vi "Methods_Insert Dividers.vi"(11 "Methods[] In":T1(array[cluster])) -> (3 "Methods[] Out":T1(array[cluster]))   [LabVIEW 2023] (continued)
"Data name"="License.Get Feature Status", "Short name (localized)"="License.Get Feature Status", "Long name (localized)"="License:Get Feature Status"}, "Method Flags"={"IsDeprecated"=FALSE, "IsPrivate"=TRUE, "IsScripting"=FALSE, "IsNotInRun-Time"=FALSE}, "Divider"=FALSE}, {"Class Info"={"Unique ID string"="1", "Parent ID string"="", "Class Name (unlocalized)"="Application", "Class Name (localized)"="Application"}, "Method Info"={"Unique ID string"="849", "Data name"="Library.Deploy Library", "Short name (localized)"="Library.Deploy Library", "Long name (localized)"="Library:Deploy Library"}, "Method Flags"={"IsDeprecated"=FALSE, "IsPrivate"=FALSE, "IsScripting"=FALSE, "IsNotInRun-Time"=FALSE}, "Divider"=FALSE}, {"Class Info"={"Unique ID string"="1", "Parent ID string"="", "Class Name (unlocalized)"="Application", "Class Name (localized)"="Application"}, "Method Info"={"Unique ID string"="84b", "Data name"="NI Sec.ChangePassword", "Short name (localized)"="NI Sec.ChangePassword", "Long name (localized)"="NI Security:Change Password"}, "Method Flags"={"IsDeprecated"=FALSE, "IsPrivate"=TRUE, "IsScripting"=FALSE, "IsNotInRun-Time"=FALSE}, "Divider"=FALSE}, {"Class Info"={"Unique ID string"="1", "Parent ID string"="", "Class Name (unlocalized)"="Application", "Class Name (localized)"="Application"}, "Method Info"={"Unique ID string"="84c", "Data name"="NI Sec.GetDomains", "Short name (localized)"="NI Sec.GetDomains", "Long name (localized)"="NI Security:Get Domains"}, "Method Flags"={"IsDeprecated"=FALSE, "IsPrivate"=TRUE, "IsScripting"=FALSE, "IsNotInRun-Time"=FALSE}, "Divider"=FALSE}, {"Class Info"={"Unique ID string"="1", "Parent ID string"="", "Class Name (unlocalized)"="Application", "Class Name (localized)"="Application"}, "Method Info"={"Unique ID string"="84d", "Data name"="Save Stock Objects", "Short name (localized)"="Save Stock Objects", "Long name (localized)"="Save Stock Objects"}, "Method Flags"={"IsDeprecated"=FALSE, "IsPrivate"=TRUE, "IsScripting"=FALSE, "IsNotInRun-Time"=TRUE}, "Divider"=FALSE}, {"Class Info"={"Unique ID string"="1", "Parent ID string"="", "Class Name (unlocalized)"="Application", "Class Name (localized)"="Application"}, "Method Info"={"Unique ID string"="84e", "Data name"="Library.UndeployLibrary", "Short name (localized)"="Library.UndeployLibrary", "Long name (localized)"="Library:Undeploy Library"}, "Method Flags"={"IsDeprecated"=FALSE, "IsPrivate"=FALSE, "IsScripting"=FALSE, "IsNotInRun-Time"=FALSE}, "Divider"=FALSE}, {"Class Info"={"Unique ID string"="1", "Parent ID string"="", "Class Name (unlocalized)"="Application", "Class Name (localized)"="Application"}, "Method Info"={"Unique ID string"="84f", "Data name"="Cmp Data Types", "Short name (localized)"="Cmp Data Types", "Long name (localized)"="Compare:Data Types"}, "Method Flags"={"IsDeprecated"=FALSE, "IsPrivate"=TRUE, "IsScripting"=FALSE, "IsNotInRun-Time"=FALSE}, "Divider"=FALSE}, {"Class Info"={"Unique ID string"="1", "Parent ID string"="", "Class Name (unlocalized)"="Application", "Class Name (localized)"="Application"}, "Method Info"={"Unique ID string"="850", "Data name"="Data Type Color", "Short name (localized)"="Data Type Color", "Long name (localized)"="Data Type Color"}, "Method Flags"={"IsDeprecated"=FALSE, "IsPrivate"=FALSE, "IsScripting"=TRUE, "IsNotInRun-Time"=FALSE}, "Divider"=FALSE}, {"Class Info"={"Unique ID string"="1", "Parent ID string"="", "Class Name (unlocalized)"="Application", "Class Name (localized)"="Application"}, "Method Info"={"Unique ID string"="851", "Data name"="Clipboard.Read", "Short name (localized)"="Clipboard.Read", "Long name (localized)"="Clipboard:Read From Clipboard"}, "Method Flags"={"IsDeprecated"=FALSE, "IsPrivate"=FALSE, "IsScripting"=FALSE, "IsNotInRun-Time"=FALSE}, "Divider"=FALSE}, {"Class Info"={"Unique ID string"="1", "Parent ID string"="", "Class Name (unlocalized)"="Application", "Class Name (localized)"="Application"}, "Method Info"={"Unique ID string"="852", "Data name"="Clipboard.Write", "Short name (localized)"="Clipboard.Write", "Long name (localized)"="Clipboard:Write to Clipboard"}, "Method Flags"={"IsDeprecated"=FALSE, "IsPrivate"=FALSE, "IsScripting"=FALSE, "IsNotInRun-Time"=FALSE}, "Divider"=FALSE}, {"Class Info"={"Unique ID string"="1", "Parent ID string"="", "Class Name (unlocalized)"="Application", "Class Name (localized)"="Application"}, "Method Info"={"Unique ID string"="853", "Data name"="RecentOpen.LVProjects", "Short name (localized)"="RecentOpen.LVProjects", "Long name (localized)"="Recently Opened:LV Projects"}, "Method Flags"={"IsDeprecated"=FALSE, "IsPrivate"=FALSE, "IsScripting"=TRUE, "IsNotInRun-Time"=TRUE}, "Divider"=FALSE}, {"Class Info"={"Unique ID string"="1", "Parent ID string"="", "Class Name (unlocalized)"="Application", "Class Name (localized)"="Application"}, "Method Info"={"Unique ID string"="854", "Data name"="Open.Recently Opened Project", "Short name (localized)"="Open.Recently Opened Project", "Long name (localized)"="Open:Recently Opened Project"}, "Method Flags"={"IsDeprecated"=FALSE, "IsPrivate"=FALSE, "IsScripting"=TRUE, "IsNotInRun-Time"=FALSE}, "Divider"=FALSE}, {"Class Info"={"Unique ID string"="1", "Parent ID string"="", "Class Name (unlocalized)"="Application", "Class Name (localized)"="Application"}, "Method Info"={"Unique ID string"="855", "Data name"="VIs Strings.Export", "Short name (localized)"="VIs Strings.Export", "Long name (localized)"="VIs Strings:Export"}, "Method Flags"={"IsDeprecated"=FALSE, "IsPrivate"=FALSE, "IsScripting"=FALSE, "IsNotInRun-Time"=TRUE}, "Divider"=FALSE}, {"Class Info"={"Unique ID string"="1", "Parent ID string"="", "Class Name (unlocalized)"="Application", "Class Name (localized)"="Application"}, "Method Info"={"Unique ID string"="856", "Data name"="VIs Strings.Import", "Short name (localized)"="VIs Strings.Import", "Long name (localized)"="VIs Strings:Import"}, "Method Flags"={"IsDeprecated"=FALSE, "IsPrivate"=FALSE, "IsScripting"=FALSE, "IsNotInRun-Time"=FALSE}, "Divider"=FALSE}, {"Class Info"={"Unique ID string"="1", "Parent ID string"="", "Class Name (unlocalized)"="Application", "Class Name (localized)"="Application"}, "Method Info"={"Unique ID string"="857", "Data name"="VIs Strings.Export Private", "Short name (localized)"="VIs Strings.Export Private", "Long name (localized)"="VIs Strings:Export Private"}, "Method Flags"={"IsDeprecated"=FALSE, "IsPrivate"=TRUE, "IsScripting"=FALSE, "IsNotInRun-Time"=TRUE}, "Divider"=FALSE}, {"Class Info"={"Unique ID string"="1", "Parent ID string"="", "Class Name (unlocalized)"="Application", "Class Name (localized)"="Application"}, "Method Info"={"Unique ID string"="858", "Data name"="Pwd.Del From Cache", "Short name (localized)"="Pwd.Del From Cache", "Long name (localized)"="Password:Delete From Cache"}, "Method Flags"={"IsDeprecated"=FALSE, "IsPrivate"=TRUE, "IsScripting"=FALSE, "IsNotInRun-Time"=FALSE}, "Divider"=FALSE}, {"Class Info"={"Unique ID string"="1", "Parent ID string"="", "Class Name (unlocalized)"="Application", "Class Name (localized)"="Application"}, "Method Info"={"Unique ID string"="859", "Data name"="LVRT.Unload Startup App", "Short name (localized)"="LVRT.Unload Startup App", "Long name (localized)"="LVRT:Unload Startup App"}, "Method Flags"={"IsDeprecated"=FALSE, "IsPrivate"=TRUE, "IsScripting"=FALSE, "IsNotInRun-Time"=TRUE}, "Divider"=FALSE}, {"Class Info"={"Unique ID string"="1", "Parent ID string"="", "Class Name (unlocalized)"="Application", "Class Name (localized)"="Application"}, "Method Info"={"Unique ID string"="85b", "Data name"="Tag.Get Tag", "Short name (localized)"="Tag.Get Tag", "Long name (localized)"="Tag:Get Tag"}, "Method Flags"={"IsDeprecated"=FALSE, "IsPrivate"=TRUE, "IsScripting"=FALSE, "IsNotInRun-Time"=FALSE}, "Divider"=FALSE}, {"Class Info"={"Unique ID string"="1", "Parent ID string"="", "Class Name (unlocalized)"="Application", "Class Name (localized)"="Application"}, "Method Info"={"Unique ID string"="85c", "Data name"="Tag.Set Tag", "Short name (localized)"="Tag.Set Tag", "Long name (localized)"="Tag:Set Tag"}, "Method Flags"={"IsDeprecated"=FALSE, "IsPrivate"=TRUE, "IsScripting"=FALSE, "IsNotInRun-Time"=FALSE}, "Divider"=FALSE}, {"Class Info"={"Unique ID string"="1", "Parent ID string"="", "Class Name (unlocalized)"="Application", "Class Name (localized)"="Application"}, "Method Info"={"Unique ID string"="85d", "Data name"="Tag.Remove All Tags", "Short name (localized)"="Tag.Remove All Tags", "Long name (localized)"="Tag:Remove All Tags"}, "Method Flags"={"IsDeprecated"=FALSE, "IsPrivate"=TRUE, "IsScripting"=FALSE, "IsNotInRun-Time"=FALSE}, "Divider"=FALSE}, {"Class Info"={"Unique ID string"="1", "Parent ID string"="", "Class Name (unlocalized)"="Application", "Class Name (localized)"="Application"}, "Method Info"={"Unique ID string"="85e", "Data name"="Tag.Remove Tag", "Short name (localized)"="Tag.Remove Tag", "Long name (localized)"="Tag:Remove Tag"}, "Method Flags"={"IsDeprecated"=FALSE, "IsPrivate"=TRUE, "IsScripting"=FALSE, "IsNotInRun-Time"=FALSE}, "Divider"=FALSE}, {"Class Info"={"Unique ID string"="1", "Parent ID string"="", "Class Name (unlocalized)"="Application", "Class Name (localized)"="Application"}, "Method Info"={"Unique ID string"="860", "Data name"="Get VI.Is Probe", "Short name (localized)"="Get VI.Is Probe", "Long name (localized)"="Get VI:Is Probe"}, "Method Flags"={"IsDeprecated"=FALSE, "IsPrivate"=FALSE, "IsScripting"=FALSE, "IsNotInRun-Time"=TRUE}, "Divider"=FALSE}, {"Class Info"={"Unique ID string"="1", "Parent ID string"="", "Class Name (unlocalized)"="Application", "Class Name (localized)"="Application"}, "Method Info"={"Unique ID string"="861", "Data name"="Refresh Palettes", "Short name (localized)"="Refresh Palettes", "Long name (localized)"="Palettes:Refresh"}, "Method Flags"={"IsDeprecated"=FALSE, "IsPrivate"=FALSE, "IsScripting"=FALSE, "IsNotInRun-Time"=TRUE}, "Divider"=FALSE}, {"Class Info"={"Unique ID string"="1", "Parent ID string"="", "Class Name (unlocalized)"="Application", "Class Name (localized)"="Application"}, "Method Info"={"Unique ID string"="862", "Data name"="GetDataTypeHelpImage", "Short name (localized)"="GetDataTypeHelpImage", "Long name (localized)"="Help Image:Get Data Type Help Image"}, "Method Flags"={"IsDeprecated"=FALSE, "IsPrivate"=TRUE, "IsScripting"=FALSE, "IsNotInRun-Time"=TRUE}, "Divider"=FALSE}, {"Class Info"={"Unique ID string"="1", "Parent ID string"="", "Class Name (unlocalized)"="Application", "Class Name (localized)"="Application"}, "Method Info"={"Unique ID string"="863", "Data name"="Context.Ref Count.Inc", "Short name (localized)"="Context.Ref Count.Inc", "Long name (localized)"="Context:Reference Count:Increment"}, "Method Flags"={"IsDeprecated"=FALSE, "IsPrivate"=TRUE, "IsScripting"=FALSE, "IsNotInRun-Time"=FALSE}, "Divider"=FALSE}, {"Class Info"={"Unique ID string"="1", "Parent ID string"="", "Class Name (unlocalized)"="Application", "Class Name (localized)"="Application"}, "Method Info"={"Unique ID string"="864", "Data name"="Context.Ref Count.Dec", "Short name (localized)"="Context.Ref Count.Dec", "Long name (localized)"="Context:Reference Count:Decrement"}, "Method Flags"={"IsDeprecated"=FALSE, "IsPrivate"=TRUE, "IsScripting"=FALSE, "IsNotInRun-Time"=FALSE}, "Divider"=FALSE}, {"Class Info"={"Unique ID string"="1", "Parent ID string"="", "Class Name (unlocalized)"="Application", "Class Name (localized)"="Application"}, "Method Info"={"Unique ID string"="865", "Data name"="NI Security.SVE Login", "Short name (localized)"="NI Security.SVE Login", "Long name (localized)"="NI Security:Shared Variable Engine Login"}, "Method Flags"={"IsDeprecated"=FALSE, "IsPrivate"=TRUE, "IsScripting"=FALSE, "IsNotInRun-Time"=FALSE}, "Divider"=FALSE}, {"Class Info"={"Unique ID string"="1", "Parent ID string"="", "Class Name (unlocalized)"="Application", "Class Name (localized)"="Application"}, "Method Info"={"Unique ID string"="866", "Data name"="NI Security.SVE Logout", "Short name (localized)"="NI Security.SVE Logout", "Long name (localized)"="NI Security:Shared Variable Engine Logout"}, "Method Flags"={"IsDeprecated"=FALSE, "IsPrivate"=TRUE, "IsScripting"=FALSE, "IsNotInRun-Time"=FALSE}, "Divider"=FALSE}, {"Class Info"={"Unique ID string"="1", "Parent ID string"="", "Class Name (unlocalized)"="Application", "Class Name (localized)"="Application"}, "Method Info"={"Unique ID string"="867", "Data name"="NI Security.SVE User", "Short name (localized)"="NI Security.SVE User", "Long name (localized)"="NI Security:Shared Variable Engine User"}, "Method Flags"={"IsDeprecated"=FALSE, "IsPrivate"=TRUE, "IsScripting"=FALSE, "IsNotInRun-Time"=FALSE}, "Divider"=FALSE}, {"Class Info"={"Unique ID string"="1", "Parent ID string"="", "Class Name (unlocalized)"="Application", "Class Name (localized)"="Application"}, "Method Info"={"Unique ID string"="868", "Data name"="Get Func Help Image", "Short name (localized)"="Get Func Help Image", "Long name (localized)"="Help Image:Get Function Context Help Image"}, "Method Flags"={"IsDeprecated"=FALSE, "IsPrivate"=TRUE, "IsScripting"=FALSE, "IsNotInRun-Time"=TRUE}, "Divider"=FALSE}, {"Class Info"={"Unique ID string"="1", "Parent ID string"="", "Class Name (unlocalized)"="Application", "Class Name (localized)"="Application"}, "Method Info"={"Unique ID string"="869", "Data name"="TD.AddPathInfo", "Short name (localized)"="TD.AddPathInfo", "Long name (localized)"="Type Descriptor:Add Path Info"}, "Method Flags"={"IsDeprecated"=FALSE, "IsPrivate"=TRUE, "IsScripting"=TRUE, "IsNotInRun-Time"=TRUE}, "Divider"=FALSE}, {"Class Info"={"Unique ID string"="1", "Parent ID string"="", "Class Name (unlocalized)"="Application", "Class Name (localized)"="Application"}, "Method Info"={"Unique ID string"="86a", "Data name"="TD.CleanPathInfo", "Short name (localized)"="TD.CleanPathInfo", "Long name (localized)"="Type Descriptor:Clean Path Info"}, "Method Flags"={"IsDeprecated"=FALSE, "IsPrivate"=TRUE, "IsScripting"=TRUE, "IsNotInRun-Time"=TRUE}, "Divider"=FALSE}, {"Class Info"={"Unique ID string"="1", "Parent ID string"="", "Class Name (unlocalized)"="Application", "Class Name (localized)"="Application"}, "Method Info"={"Unique ID string"="86b", "Data name"="TD.RecTypedefDisconnect", "Short name (localized)"="TD.RecTypedefDisconnect", "Long name (localized)"="Type Descriptor:Recursive Typedef Disconnect"}, "Method Flags"={"IsDeprecated"=FALSE, "IsPrivate"=TRUE, "IsScripting"=TRUE, "IsNotInRun-Time"=TRUE}, "Divider"=FALSE}, {"Class Info"={"Unique ID string"="1", "Parent ID string"="", "Class Name (unlocalized)"="Application", "Class Name (localized)"="Application"}, "Method Info"={"Unique ID string"="86c", "Data name"="GetClassNameFromID", "Short name (localized)"="GetClassNameFromID", "Long name (localized)"="Get Class Name From Class ID"}, "Method Flags"={"IsDeprecated"=FALSE, "IsPrivate"=TRUE, "IsScripting"=FALSE, "IsNotInRun-Time"=FALSE}, "Divider"=FALSE}, {"Class Info"={"Unique ID string"="1", "Parent ID string"="", "Class Name (unlocalized)"="Application", "Class Name (localized)"="Application"}, "Method Info"={"Unique ID string"="86d", "Data name"="Context.GetFromProj", "Short name (localized)"="Context.GetFromProj", "Long name (localized)"="Context:Get From Project"}, "Method Flags"={"IsDeprecated"=FALSE, "IsPrivate"=TRUE, "IsScripting"=FALSE, "IsNotInRun-Time"=TRUE}, "Divider"=FALSE}, {"Class Info"={"Unique ID string"="1", "Parent ID string"="", "Class Name (unlocalized)"="Application", "Class Name (localized)"="Application"}, "Method Info"={"Unique ID string"="86e", "Data name"="Library.GetFileLVVersion", "Short name (localized)"="Library.GetFileLVVersion", "Long name (localized)"="Library:Get File LabVIEW Version"}, "Method Flags"={"IsDeprecated"=FALSE, "IsPrivate"=FALSE, "IsScripting"=FALSE, "IsNotInRun-Time"=FALSE}, "Divider"=FALSE}, {"Class Info"={"Unique ID string"="1", "Parent ID string"="", "Class Name (unlocalized)"="Application", "Class Name (localized)"="Application"}, "Method Info"={"Unique ID string"="86f", "Data name"="TD.HasCompletePathInfo", "Short name (localized)"="TD.HasCompletePathInfo", "Long name (localized)"="Type Descriptor:Has Complete Path Info"}, "Method Flags"={"IsDeprecated"=FALSE, "IsPrivate"=TRUE, "IsScripting"=TRUE, "IsNotInRun-Time"=TRUE}, "Divider"=FALSE}, {"Class Info"={"Unique ID string"="1", "Parent ID string"="", "Class Name (unlocalized)"="Application", "Class Name (localized)"="Application"}, "Method Info"={"Unique ID string"="870", "Data name"="Add To MRU", "Short name (localized)"="Add To MRU", "Long name (localized)"="Add To Most Recently Used List"}, "Method Flags"={"IsDeprecated"=FALSE, "IsPrivate"=TRUE, "IsScripting"=FALSE, "IsNotInRun-Time"=FALSE}, "Divider"=FALSE}, {"Class Info"={"Unique ID string"="1", "Parent ID string"="", "Class Name (unlocalized)"="Application", "Class Name (localized)"="Application"}, "Method Info"={"Unique ID string"="871", "Data name"="Project.OpenPrivCtxts", "Short name (localized)"="Project.OpenPrivCtxts", "Long name (localized)"="Project:Open With Private Contexts"}, "Method Flags"={"IsDeprecated"=FALSE, "IsPrivate"=TRUE, "IsScripting"=FALSE, "IsNotInRun-Time"=FALSE}, "Divider"=FALSE}, {"Class Info"={"Unique ID string"="1", "Parent ID string"="", "Class Name (unlocalized)"="Application", "Class Name (localized)"="Application"}, "Method Info"={"Unique ID string"="872", "Data name"="LVRT.Transfer Files", "Short name (localized)"="LVRT.Transfer Files", "Long name (localized)"="LVRT:Transfer Files To Target"}, "Method Flags"={"IsDeprecated"=FALSE, "IsPrivate"=TRUE, "IsScripting"=FALSE, "IsNotInRun-Time"=TRUE}, "Divider"=FALSE}, {"Class Info"={"Unique ID string"="1", "Parent ID string"="", "Class Name (unlocalized)"="Application", "Class Name (localized)"="Application"}, "Method Info"={"Unique ID string"="873", "Data name"="Scene.New Object", "Short name (localized)"="Scene.New Object", "Long name (localized)"="Scene:New Object"}, "Method Flags"={"IsDeprecated"=FALSE, "IsPrivate"=FALSE, "IsScripting"=FALSE, "IsNotInRun-Time"=FALSE}, "Divider"=FALSE}, {"Class Info"={"Unique ID string"="1", "Parent ID string"="", "Class Name (unlocalized)"="Application", "Class Name (localized)"="Application"}, "Method Info"={"Unique ID string"="874", "Data name"="Scene.New Texture", "Short name (localized)"="Scene.New Texture", "Long name (localized)"="Scene:New Texture"}, "Method Flags"={"IsDeprecated"=FALSE, "IsPrivate"=FALSE, "IsScripting"=FALSE, "IsNotInRun-Time"=FALSE}, "Divider"=FALSE}, {"Class Info"={"Unique ID string"="1", "Parent ID string"="", "Class Name (unlocalized)"="Application", "Class Name (localized)"="Application"}, "Method Info"={"Unique ID string"="877", "Data name"="Scene.Drawable.Geometry.New Box", "Short name (localized)"="Scene.Drawable.Geometry.New Box", "Long name (localized)"="Scene:Drawable:Geometry:New Box"}, "Method Flags"={"IsDeprecated"=FALSE, "IsPrivate"=FALSE, "IsScripting"=FALSE, "IsNotInRun-Time"=FALSE}, "Divider"=FALSE}, {"Class Info"={"Unique ID string"="1", "Parent ID string"="", "Class Name (unlocalized)"="Application", "Class Name (localized)"="Application"}, "Method Info"={"Unique ID string"="878", "Data name"="Scene.Drawable.Geometry.New Cone", "Short name (localized)"="Scene.Drawable.Geometry.New Cone", "Long name (localized)"="Scene:Drawable:Geometry:New Cone"}, "Method Flags"={"IsDeprecated"=FALSE, "IsPrivate"=FALSE, "IsScripting"=FALSE, "IsNotInRun-Time"=FALSE}, "Divider"=FALSE}, {"Class Info"={"Unique ID string"="1", "Parent ID string"="", "Class Name (unlocalized)"="Application", "Class Name (localized)"="Application"}, "Method Info"={"Unique ID string"="879", "Data name"="Scene.Drawable.Geometry.New Cylinder", "Short name (localized)"="Scene.Drawable.Geometry.New Cylinder", "Long name (localized)"="Scene:Drawable:Geometry:New Cylinder"}, "Method Flags"={"IsDeprecated"=FALSE, "IsPrivate"=FALSE, "IsScripting"=FALSE, "IsNotInRun-Time"=FALSE}, "Divider"=FALSE}, {"Class Info"={"Unique ID string"="1", "Parent ID string"="", "Class Name (unlocalized)"="Application", "Class Name (localized)"="Application"}, "Method Info"={"Unique ID string"="87a", "Data name"="Scene.Drawable.Geometry.New Height Field", "Short name (localized)"="Scene.Drawable.Geometry.New Height Field", "Long name (localized)"="Scene:Drawable:Geometry:New Height Field"}, "Method Flags"={"IsDeprecated"=FALSE, "IsPrivate"=FALSE, "IsScripting"=FALSE, "IsNotInRun-Time"=FALSE}, "Divider"=FALSE}, {"Class Info"={"Unique ID string"="1", "Parent ID string"="", "Class Name (unlocalized)"="Application", "Class Name (localized)"="Application"}, "Method Info"={"Unique ID string"="87b", "Data name"="Scene.Drawable.Geometry.New Sphere", "Short name (localized)"="Scene.Drawable.Geometry.New Sphere", "Long name (localized)"="Scene:Drawable:Geometry:New Sphere"}, "Method Flags"={"IsDeprecated"=FALSE, "IsPrivate"=FALSE, "IsScripting"=FALSE, "IsNotInRun-Time"=FALSE}, "Divider"=FALSE}, {"Class Info"={"Unique ID string"="1", "Parent ID string"="", "Class Name (unlocalized)"="Application", "Class Name (localized)"="Application"}, "Method Info"={"Unique ID string"="87c", "Data name"="Scene.Drawable.Geometry.New Mesh", "Short name (localized)"="Scene.Drawable.Geometry.New Mesh", "Long name (localized)"="Scene:Drawable:Geometry:New Mesh"}, "Method Flags"={"IsDeprecated"=FALSE, "IsPrivate"=FALSE, "IsScripting"=FALSE, "IsNotInRun-Time"=FALSE}, "Divider"=FALSE}, {"Class Info"={"Unique ID string"="1", "Parent ID string"="", "Class Name (unlocalized)"="Application", "Class Name (localized)"="Application"}, "Method Info"={"Unique ID string"="87e", "Data name"="Scene.New Clip Plane", "Short name (localized)"="Scene.New Clip Plane", "Long name (localized)"="Scene:New Clip Plane"}, "Method Flags"={"IsDeprecated"=FALSE, "IsPrivate"=FALSE, "IsScripting"=FALSE, "IsNotInRun-Time"=FALSE}, "Divider"=FALSE}, {"Class Info"={"Unique ID string"="1", "Parent ID string"="", "Class Name (unlocalized)"="Application", "Class Name (localized)"="Application"}, "Method Info"={"Unique ID string"="87f", "Data name"="Scene.New Window", "Short name (localized)"="Scene.New Window", "Long name (localized)"="Scene:New Window"}, "Method Flags"={"IsDeprecated"=FALSE, "IsPrivate"=FALSE, "IsScripting"=FALSE, "IsNotInRun-Time"=FALSE}, "Divider"=FALSE}, {"Class Info"={"Unique ID string"="1", "Parent ID string"="", "Class Name (unlocalized)"="Application", "Class Name (localized)"="Application"}, "Method Info"={"Unique ID string"="880", "Data name"="Scene.Write Scene File", "Short name (localized)"="Scene.Write Scene File", "Long name (localized)"="Scene:Write Scene File"}, "Method Flags"={"IsDeprecated"=FALSE, "IsPrivate"=FALSE, "IsScripting"=FALSE, "IsNotInRun-Time"=FALSE}, "Divider"=FALSE}, {"Class Info"={"Unique ID string"="1", "Parent ID string"="", "Class Name (unlocalized)"="Application", "Class Name (localized)"="Application"}, "Method Info"={"Unique ID string"="881", "Data name"="Scene.Read Scene File", "Short name (localized)"="Scene.Read Scene File", "Long name (localized)"="Scene:Read Scene File"}, "Method Flags"={"IsDeprecated"=FALSE, "IsPrivate"=FALSE, "IsScripting"=FALSE, "IsNotInRun-Time"=FALSE}, "Divider"=FALSE}, {"Class Info"={"Unique ID string"="1", "Parent ID string"="", "Class Name (unlocalized)"="Application", "Class Name (localized)"="Application"}, "Method Info"={"Unique ID string"="882", "Data name"="ForceAutoSave", "Short name (localized)"="ForceAutoSave", "Long name (localized)"="Force AutoSave"}, "Method Flags"={"IsDeprecated"=FALSE, "IsPrivate"=TRUE, "IsScripting"=FALSE, "IsNotInRun-Time"=TRUE}, "Divider"=FALSE}, {"Class Info"={"Unique ID string"="1", "Parent ID string"="", "Class Name (unlocalized)"="Application", "Class Name (localized)"="Application"}, "Method Info"={"Unique ID string"="883", "Data name"=".NET.Load Assembly", "Short name (localized)"=".NET.Load Assembly", "Long name (localized)"=".NET:Load Assembly To ObjMgr"}, "Method Flags"={"IsDeprecated"=FALSE, "IsPrivate"=TRUE, "IsScripting"=TRUE, "IsNotInRun-Time"=TRUE}, "Divider"=FALSE}, {"Class Info"={"Unique ID string"="1", "Parent ID string"="", "Class Name (unlocalized)"="Application", "Class Name (localized)"="Application"}, "Method Info"={"Unique ID string"="884", "Data name"="Get VI Tag", "Short name (localized)"="Get VI Tag", "Long name (localized)"="Tag:VI:Get VI Tag"}, "Method Flags"={"IsDeprecated"=FALSE, "IsPrivate"=TRUE, "IsScripting"=FALSE, "IsNotInRun-Time"=FALSE}, "Divider"=FALSE}, {"Class Info"={"Unique ID string"="1", "Parent ID string"="", "Class Name (unlocalized)"="Application", "Class Name (localized)"="Application"}, "Method Info"={"Unique ID string"="885", "Data name"="Set VI Tag", "Short name (localized)"="Set VI Tag", "Long name (localized)"="Tag:VI:Set VI Tag"}, "Method Flags"={"IsDeprecated"=FALSE, "IsPrivate"=TRUE, "IsScripting"=FALSE, "IsNotInRun-Time"=TRUE}, "Divider"=FALSE}, {"Class Info"={"Unique ID string"="1", "Parent ID string"="", "Class Name (unlocalized)"="Application", "Class Name (localized)"="Application"}, "Method Info"={"Unique ID string"="886", "Data name"="Get VI.Revision History", "Short name (localized)"="Get VI.Revision History", "Long name (localized)"="Get VI:Revision History"}, "Method Flags"={"IsDeprecated"=FALSE, "IsPrivate"=FALSE, "IsScripting"=FALSE, "IsNotInRun-Time"=FALSE}, "Divider"=FALSE}, {"Class Info"={"Unique ID string"="1", "Parent ID string"="", "Class Name (unlocalized)"="Application", "Class Name (localized)"="Application"}, "Method Info"={"Unique ID string"="887", "Data name"="Sig.GetUserCodeGUIDFromVIFile", "Short name (localized)"="Sig.GetUserCodeGUIDFromVIFile", "Long name (localized)"="Signature:Get User Code GUID From VI File"}, "Method Flags"={"IsDeprecated"=FALSE, "IsPrivate"=TRUE, "IsScripting"=FALSE, "IsNotInRun-Time"=FALSE}, "Divider"=FALSE}, {"Class Info"={"Unique ID string"="1", "Parent ID string"="", "Class Name (unlocalized)"="Application", "Class Name (localized)"="Application"}, "Method Info"={"Unique ID string"="888", "Data name"="Sig.GetSignatureFromVIFile", "Short name (localized)"="Sig.GetSignatureFromVIFile", "Long name (localized)"="Signature:Get Signature From VI File"}, "Method Flags"={"IsDeprecated"=FALSE, "IsPrivate"=TRUE, "IsScripting"=FALSE, "IsNotInRun-Time"=FALSE}, "Divider"=FALSE}, {"Class Info"={"Unique ID string"="1", "Parent ID string"="", "Class Name (unlocalized)"="Application", "Class Name (localized)"="Application"}, "Method Info"={"Unique ID string"="889", "Data name"="Scene.New Light", "Short name (localized)"="Scene.New Light", "Long name (localized)"="Scene:New Light"}, "Method Flags"={"IsDeprecated"=FALSE, "IsPrivate"=FALSE, "IsScripting"=FALSE, "IsNotInRun-Time"=FALSE}, "Divider"=FALSE}, {"Class Info"={"Unique ID string"="1", "Parent ID string"="", "Class Name (unlocalized)"="Application", "Class Name (localized)"="Application"}, "Method Info"={"Unique ID string"="88a", "Data name"="Update Launch Message", "Short name (localized)"="Update Launch Message", "Long name (localized)"="Update Launch Message"}, "Method Flags"={"IsDeprecated"=FALSE, "IsPrivate"=TRUE, "IsScripting"=FALSE, "IsNotInRun-Time"=FALSE}, "Divider"=FALSE}, {"Class Info"={"Unique ID string"="1", "Parent ID string"="", "Class Name (unlocalized)"="Application", "Class Name (localized)"="Application"}, "Method Info"={"Unique ID string"="88b", "Data name"="BitAccurateDataSizeForType", "Short name (localized)"="BitAccurateDataSizeForType", "Long name (localized)"="Bit Accurate Data Size For Type"}, "Method Flags"={"IsDeprecated"=FALSE, "IsPrivate"=TRUE, "IsScripting"=TRUE, "IsNotInRun-Time"=FALSE}, "Divider"=FALSE}, {"Class Info"={"Unique ID string"="1", "Parent ID string"="", "Class Name (unlocalized)"="Application", "Class Name (localized)"="Application"}, "Method Info"={"Unique ID string"="88c", "Data name"="Get VI.Icon", "Short name (localized)"="Get VI.Icon", "Long name (localized)"="Get VI:Icon"}, "Method Flags"={"IsDeprecated"=FALSE, "IsPrivate"=FALSE, "IsScripting"=FALSE, "IsNotInRun-Time"=FALSE}, "Divider"=FALSE}, {"Class Info"={"Unique ID string"="1", "Parent ID string"="", "Class Name (unlocalized)"="Application", "Class Name (localized)"="Application"}, "Method Info"={"Unique ID string"="88d", "Data name"="Notify LV SCC Enabled", "Short name (localized)"="Notify LV SCC Enabled", "Long name (localized)"="Notify LV SCC Enabled"}, "Method Flags"={"IsDeprecated"=FALSE, "IsPrivate"=TRUE, "IsScripting"=FALSE, "IsNotInRun-Time"=FALSE}, "Divider"=FALSE}, {"Class Info"={"Unique ID string"="1", "Parent ID string"="", "Class Name (unlocalized)"="Application", "Class Name (localized)"="Application"}, "Method Info"={"Unique ID string"="88e", "Data name"="LVClass.Open", "Short name (localized)"="LVClass.Open", "Long name (localized)"="LabVIEW Class:Open"}, "Method Flags"={"IsDeprecated"=FALSE, "IsPrivate"=FALSE, "IsScripting"=FALSE, "IsNotInRun-Time"=TRUE}, "Divider"=FALSE}, {"Class Info"={"Unique ID string"="1", "Parent ID string"="", "Class Name (unlocalized)"="Application", "Class Name (localized)"="Application"}, "Method Info"={"Unique ID string"="88f", "Data name"="LVClass.Create", "Short name (localized)"="LVClass.Create", "Long name (localized)"="LabVIEW Class:Create"}, "Method Flags"={"IsDeprecated"=FALSE, "IsPrivate"=FALSE, "IsScripting"=FALSE, "IsNotInRun-Time"=TRUE}, "Divider"=FALSE}, {"Class Info"={"Unique ID string"="1", "Parent ID string"="", "Class Name (unlocalized)"="Application", "Class Name (localized)"="Application"}, "Method Info"={"Unique ID string"="890", "Data name"="SyncEverything", "Short name (localized)"="SyncEverything", "Long name (localized)"="Synchronize Everything"}, "Method Flags"={"IsDeprecated"=FALSE, "IsPrivate"=TRUE, "IsScripting"=FALSE, "IsNotInRun-Time"=FALSE}, "Divider"=FALSE}, {"Class Info"={"Unique ID string"="1", "Parent ID string"="", "Class Name (unlocalized)"="Application", "Class Name (localized)"="Application"}, "Method Info"={"Unique ID string"="893", "Data name"="Project.Close Refs", "Short name (localized)"="Project.Close Refs", "Long name (localized)"="Project:Close Refs"}, "Method Flags"={"IsDeprecated"=FALSE, "IsPrivate"=TRUE, "IsScripting"=FALSE, "IsNotInRun-Time"=FALSE}, "Divider"=FALSE}, {"Class Info"={"Unique ID string"="1", "Parent ID string"="", "Class Name (unlocalized)"="Application", "Class Name (localized)"="Application"}, "Method Info"={"Unique ID string"="894", "Data name"="UI.Merge VIs", "Short name (localized)"="UI.Merge VIs", "Long name (localized)"="User Interaction:Merge VIs"}, "Method Flags"={"IsDeprecated"=FALSE, "IsPrivate"=TRUE, "IsScripting"=FALSE, "IsNotInRun-Time"=TRUE}, "Divider"=FALSE}, {"Class Info"={"Unique ID string"="1", "Parent ID string"="", "Class Name (unlocalized)"="Application", "Class Name (localized)"="Application"}, "Method Info"={"Unique ID string"="895", "Data name"="Library.Deploy Libraries", "Short name (localized)"="Library.Deploy Libraries", "Long name (localized)"="Library:Deploy Libraries"}, "Method Flags"={"IsDeprecated"=FALSE, "IsPrivate"=FALSE, "IsScripting"=FALSE, "IsNotInRun-Time"=FALSE}, "Divider"=FALSE}, {"Class Info"={"Unique ID string"="1", "Parent ID string"="", "Class Name (unlocalized)"="Application", "Class Name (localized)"="Application"}, "Method Info"={"Unique ID string"="896", "Data name"="Get VI Tag Names", "Short name (localized)"="Get VI Tag Names", "Long name (localized)"="Tag:VI:Get VI Tag Names"}, "Method Flags"={"IsDeprecated"=FALSE, "IsPrivate"=TRUE, "IsScripting"=FALSE, "IsNotInRun-Time"=FALSE}, "Divider"=FALSE}, {"Class Info"={"Unique ID string"="1", "Parent ID string"="", "Class Name (unlocalized)"="Application", "Class Name (localized)"="Application"}, "Method Info"={"Unique ID string"="897", "Data name"="Statechart.Open", "Short name (localized)"="Statechart.Open", "Long name (localized)"="Statechart:Open"}, "Method Flags"={"IsDeprecated"=FALSE, "IsPrivate"=FALSE, "IsScripting"=FALSE, "IsNotInRun-Time"=TRUE}, "Divider"=FALSE}, {"Class Info"={"Unique ID string"="1", "Parent ID string"="", "Class Name (unlocalized)"="Application", "Class Name (localized)"="Application"}, "Method Info"={"Unique ID string"="898", "Data name"="Statechart.Create", "Short name (localized)"="Statechart.Create", "Long name (localized)"="Statechart:Create"}, "Method Flags"={"IsDeprecated"=FALSE, "IsPrivate"=FALSE, "IsScripting"=FALSE, "IsNotInRun-Time"=TRUE}, "Divider"=FALSE}, {"Class Info"={"Unique ID string"="1", "Parent ID string"="", "Class Name (unlocalized)"="Application", "Class Name (localized)"="Application"}, "Method Info"={"Unique ID string"="899", "Data name"="Project.OpenAsUntitled", "Short name (localized)"="Project.OpenAsUntitled", "Long name (localized)"="Project:Open As Untitled"}, "Method Flags"={"IsDeprecated"=FALSE, "IsPrivate"=TRUE, "IsScripting"=FALSE, "IsNotInRun-Time"=TRUE}, "Divider"=FALSE}, {"Class Info"={"Unique ID string"="1", "Parent ID string"="", "Class Name (unlocalized)"="Application", "Class Name (localized)"="Application"}, "Method Info"={"Unique ID string"="89a", "Data name"="Library.OpenAsUntitled", "Short name (localized)"="Library.OpenAsUntitled", "Long name (localized)"="Library:OpenAsUntitled"}, "Method Flags"={"IsDeprecated"=FALSE, "IsPrivate"=TRUE, "IsScripting"=FALSE, "IsNotInRun-Time"=TRUE}, "Divider"=FALSE}, {"Class Info"={"Unique ID string"="1", "Parent ID string"="", "Class Name (unlocalized)"="Application", "Class Name (localized)"="Application"}, "Method Info"={"Unique ID string"="89b", "Data name"="DebugStartTiming", "Short name (localized)"="DebugStartTiming", "Long name (localized)"="Debug Start Timing"}, "Method Flags"={"IsDeprecated"=FALSE, "IsPrivate"=TRUE, "IsScripting"=FALSE, "IsNotInRun-Time"=FALSE}, "Divider"=FALSE}, {"Class Info"={"Unique ID string"="1", "Parent ID string"="", "Class Name (unlocalized)"="Application", "Class Name (localized)"="Application"}, "Method Info"={"Unique ID string"="89c", "Data name"="Linker.Read Info From File", "Short name (localized)"="Linker.Read Info From File", "Long name (localized)"="Linker:Read Info From File"}, "Method Flags"={"IsDeprecated"=FALSE, "IsPrivate"=TRUE, "IsScripting"=FALSE, "IsNotInRun-Time"=TRUE}, "Divider"=FALSE}, {"Class Info"={"Unique ID string"="1", "Parent ID string"="", "Class Name (unlocalized)"="Application", "Class Name (localized)"="Application"}, "Method Info"={"Unique ID string"="89d", "Data name"="OpenErrWdw", "Short name (localized)"="OpenErrWdw", "Long name (localized)"="Error Window:Open"}, "Method Flags"={"IsDeprecated"=FALSE, "IsPrivate"=TRUE, "IsScripting"=FALSE, "IsNotInRun-Time"=FALSE}, "Divider"=FALSE}, {"Class Info"={"Unique ID string"="1", "Parent ID string"="", "Class Name (unlocalized)"="Application", "Class Name (localized)"="Application"}, "Method Info"={"Unique ID string"="89e", "Data name"="DbgConn.GetDbgConn", "Short name (localized)"="DbgConn.GetDbgConn", "Long name (localized)"="Debug Connection:Get Debug Connection"}, "Method Flags"={"IsDeprecated"=FALSE, "IsPrivate"=TRUE, "IsScripting"=FALSE, "IsNotInRun-Time"=TRUE}, "Divider"=FALSE}, {"Class Info"={"Unique ID string"="1", "Parent ID string"="", "Class Name (unlocalized)"="Application", "Class Name (localized)"="Application"}, "Method Info"={"Unique ID string"="89f", "Data name"="CreateGUID", "Short name (localized)"="CreateGUID", "Long name (localized)"="Create GUID"}, "Method Flags"={"IsDeprecated"=FALSE, "IsPrivate"=TRUE, "IsScripting"=FALSE, "IsNotInRun-Time"=FALSE}, "Divider"=FALSE}, {"Class Info"={"Unique ID string"="1", "Parent ID string"="", "Class Name (unlocalized)"="Application", "Class Name (localized)"="Application"}, "Method Info"={"Unique ID string"="900", "Data name"="Scene.Drawable.New Text", "Short name (localized)"="Scene.Drawable.New Text", "Long name (localized)"="Scene:Drawable:New Text"}, "Method Flags"={"IsDeprecated"=FALSE, "IsPrivate"=FALSE, "IsScripting"=FALSE, "IsNotInRun-Time"=FALSE}, "Divider"=FALSE}, {"Class Info"={"Unique ID string"="1", "Parent ID string"="", "Class Name (unlocalized)"="Application", "Class Name (localized)"="Application"}, "Method Info"={"Unique ID string"="901", "Data name"="OpenVIAsTemplate", "Short name (localized)"="OpenVIAsTemplate", "Long name (localized)"="Open:VI As Template"}, "Method Flags"={"IsDeprecated"=FALSE, "IsPrivate"=TRUE, "IsScripting"=FALSE, "IsNotInRun-Time"=FALSE}, "Divider"=FALSE}, {"Class Info"={"Unique ID string"="1", "Parent ID string"="", "Class Name (unlocalized)"="Application", "Class Name (localized)"="Application"}, "Method Info"={"Unique ID string"="902", "Data name"="ForceUpdateDiskMonitoring", "Short name (localized)"="ForceUpdateDiskMonitoring", "Long name (localized)"="Force Update Disk Monitoring"}, "Method Flags"={"IsDeprecated"=FALSE, "IsPrivate"=TRUE, "IsScripting"=FALSE, "IsNotInRun-Time"=FALSE}, "Divider"=FALSE}, {"Class Info"={"Unique ID string"="1", "Parent ID string"="", "Class Name (unlocalized)"="Application", "Class Name (localized)"="Application"}, "Method Info"={"Unique ID string"="903", "Data name"="MultiPwdPromptOperation.Begin", "Short name (localized)"="MultiPwdPromptOperation.Begin", "Long name (localized)"="Multi Pwd Prompt Operation:Begin"}, "Method Flags"={"IsDeprecated"=FALSE, "IsPrivate"=TRUE, "IsScripting"=TRUE, "IsNotInRun-Time"=TRUE}, "Divider"=FALSE}, {"Class Info"={"Unique ID string"="1", "Parent ID string"="", "Class Name (unlocalized)"="Application", "Class Name (localized)"="Application"}, "Method Info"={"Unique ID string"="904", "Data name"="MultiPwdPromptOperation.End", "Short name (localized)"="MultiPwdPromptOperation.End", "Long name (localized)"="Multi Pwd Prompt Operation:End"}, "Method Flags"={"IsDeprecated"=FALSE, "IsPrivate"=TRUE, "IsScripting"=TRUE, "IsNotInRun-Time"=TRUE}, "Divider"=FALSE}, {"Class Info"={"Unique ID string"="1", "Parent ID string"="", "Class Name (unlocalized)"="Application", "Class Name (localized)"="Application"}, "Method Info"={"Unique ID string"="905", "Data name"="DTT.Setup", "Short name (localized)"="DTT.Setup", "Long name (localized)"="Desktop Tracing:Setup"}, "Method Flags"={"IsDeprecated"=FALSE, "IsPrivate"=TRUE, "IsScripting"=FALSE, "IsNotInRun-Time"=FALSE}, "Divider"=FALSE}, {"Class Info"={"Unique ID string"="1", "Parent ID string"="", "Class Name (unlocalized)"="Application", "Class Name (localized)"="Application"}, "Method Info"={"Unique ID string"="906", "Data name"="DTT.GetTraceData", "Short name (localized)"="DTT.GetTraceData", "Long name (localized)"="Desktop Tracing:Get Trace Data"}, "Method Flags"={"IsDeprecated"=FALSE, "IsPrivate"=TRUE, "IsScripting"=FALSE, "IsNotInRun-Time"=FALSE}, "Divider"=FALSE}, {"Class Info"={"Unique ID string"="1", "Parent ID string"="", "Class Name (unlocalized)"="Application", "Class Name (localized)"="Application"}, "Method Info"={"Unique ID string"="909", "Data name"="Get Global Dependency Data", "Short name (localized)"="Get Global Dependency Data", "Long name (localized)"="Get Global Dependency Data"}, "Method Flags"={"IsDeprecated"=FALSE, "IsPrivate"=TRUE, "IsScripting"=FALSE, "IsNotInRun-Time"=FALSE}, "Divider"=FALSE}, {"Class Info"={"Unique ID string"="1", "Parent ID string"="", "Class Name (unlocalized)"="Application", "Class Name (localized)"="Application"}, "Method Info"={"Unique ID string"="90a", "Data name"="Invalidate Depdendency File Info", "Short name (localized)"="Invalidate Depdendency File Info", "Long name (localized)"="Invalidate Depdendency File Info"}, "Method Flags"={"IsDeprecated"=FALSE, "IsPrivate"=TRUE, "IsScripting"=FALSE, "IsNotInRun-Time"=FALSE}, "Divider"=FALSE}, {"Class Info"={"Unique ID string"="1", "Parent ID string"="", "Class Name (unlocalized)"="Application", "Class Name (localized)"="Application"}, "Method Info"={"Unique ID string"="90b", "Data name"="Project.Register Debug VI", "Short name (localized)"="Project.Register Debug VI", "Long name (localized)"="Project:Register Debug VI"}, "Method Flags"={"IsDeprecated"=FALSE, "IsPrivate"=TRUE, "IsScripting"=FALSE, "IsNotInRun-Time"=FALSE}, "Divider"=FALSE}, {"Class Info"={"Unique ID string"="1", "Parent ID string"="", "Class 
